vi "WSVCAP SHL Host TL RFFE Write.vi"(0 "RFFE Data Out":u8[][](array[numeric]) format="%.0x", 5 "Socket Mask":u64=1 format="%016x", 11 "error in":errorcluster, 13 "Log (T)":bool=TRUE, 14 "FPGA":T1) -> (15 "error out":errorcluster)   [LabVIEW 2017]
uses:
  Type Defs/WSVCAP SHL FPGA Enum.ctl
  Type Defs/WSVCAP SHL Function Enum.ctl
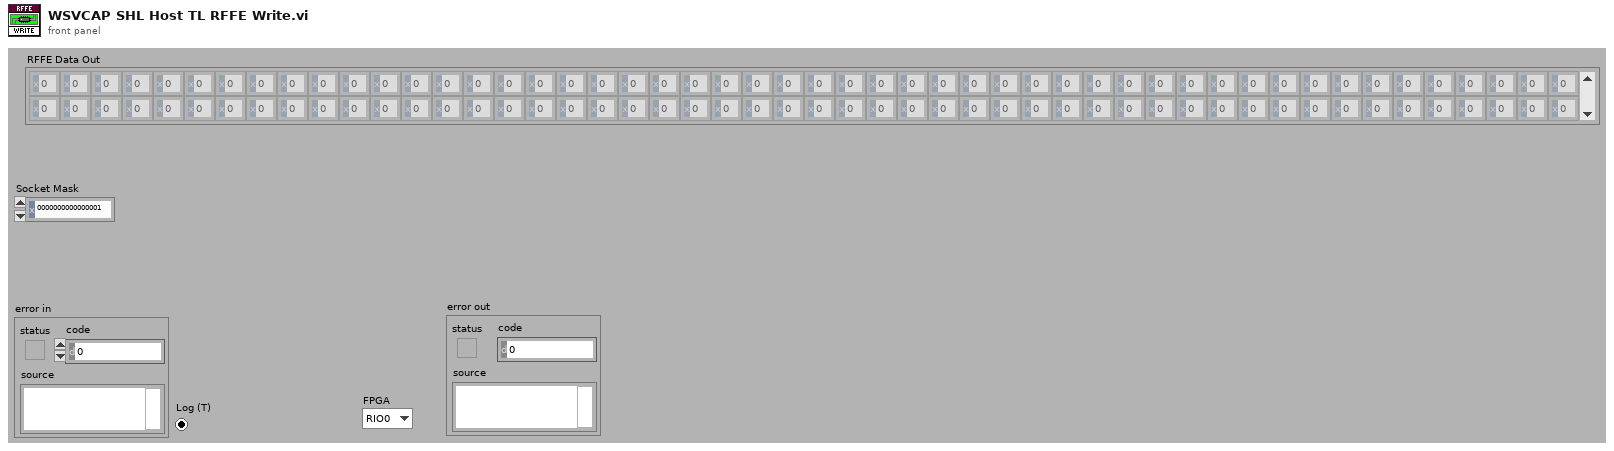
[diagram p1: front panel]
types:
  T1 = typedef "WSVCAP SHL FPGA Enum.ctl" = enum16{"RIO0", "RIO1"}
  T2 = typedef "WSVCAP SHL Function Enum.ctl" = enum16{"Initialize", "Configure I2C", "Configure RFFE", "Write I2C", "Read I2C", "Write RFFE", "Read RFFE", "Start RFFE Cycle", "Stop RFFE Cycle", "Get Status", "Close"}
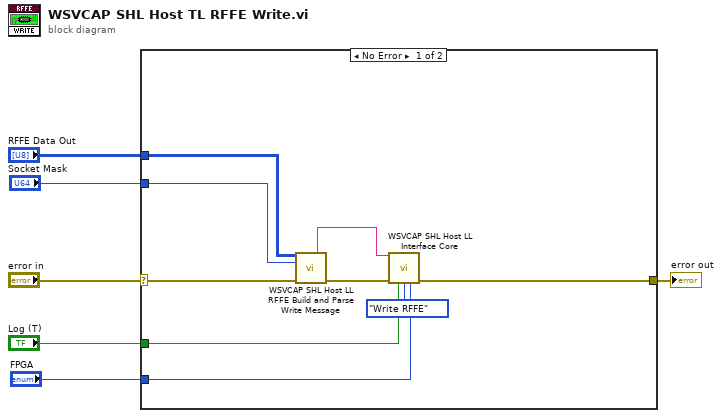
[diagram p0: block diagram]
diagram:
  n1 = case shown="No Error" "error in" {
    selector: "error in" -> [w12 w16]
    tunnel: [w8 w16] -> w6
    tunnel: "RFFE Data Out" -> [w11 _]
    tunnel: "Socket Mask" -> [w9 _]
    tunnel: "Log (T)" -> [w10 _]
    tunnel: "FPGA" -> [w7 _]
    frame No Error {
      n2 = call "WSVCAP SHL Host LL RFFE Build and Parse Write Message.vi"("Write Data In [DUT Ordered]"=w11, "Socket Mask [U64] In"=w9, "error in"=w12) -> ("Message Out"=w13:string, "error out"=w14:errorcluster)  [unwired: 6 in, 5 out]
      n3 = call "WSVCAP SHL Host LL Interface Core.vi"("Message In"=w13, "error in"=w14, "Log (T)"=w10, "Function"=WSVCAP_SHL_Function_Enum."Write RFFE", "FPGA"=w7) -> ("error out"=w8:errorcluster)  [unwired: 8 in, 2 out]
    }
    frame Error {
    }
  }
  "error out" <- w6
